vi "数据包生成.vi"(0 "状态：":string, 1 "旋转角度：":dbl, 2 "脉冲频率：":dbl, 3 "旋转方向：":bool, 4 "帧头：":string) -> (5 "数据包":string)   [LabVIEW 2018]
panel:
  out "旋转频率字符串":string
  out "旋转频率长度字符串":string
  out "旋转角度":string
  out "旋转角度字长字符串":string
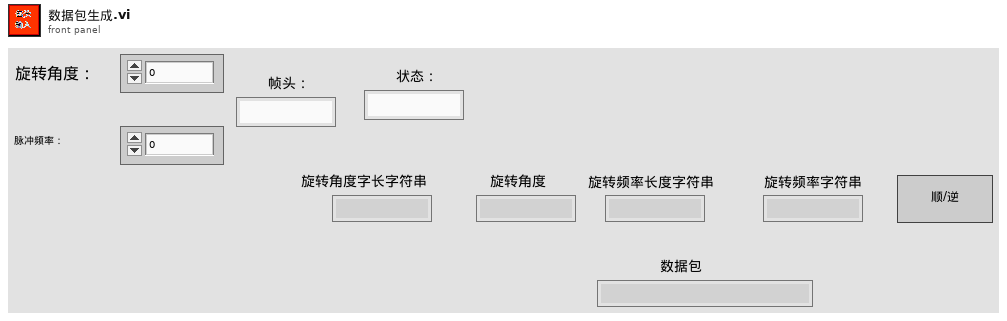
[diagram p1: front panel]
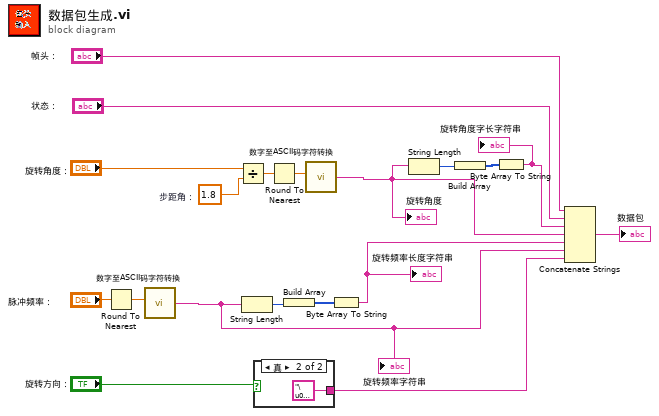
[diagram p0: block diagram]
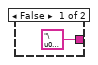
[diagram p2: hidden frame]
diagram:
  w19 = 1.8  # 步距角：
  n1 = Round To Nearest(number="脉冲频率：") -> (nearest integer value=w7:dbl)
  n2 = call "数字至ASCII码字符转换.vi"("数字"=w7) -> ("ASCII码字符串"=w1:string)  [unwired: 3 in]
  "旋转频率字符串" <- w1
  n3 = Divide(x="旋转角度：", y=w19) -> (x/y=w17:dbl)
  n4 = String Length(string=w1) -> (length=w9:i32)
  n5 = case shown="真" "旋转方向：" {
    tunnel: ["\u0000" "\u0001"] -> w6
    frame False {
    }
    frame True {
    }
  }
  n6 = Round To Nearest(number=w17) -> (nearest integer value=w8:dbl)
  n7 = Build Array(w9) -> (w10:i32[])
  n8 = call "数字至ASCII码字符转换.vi"("数字"=w8) -> ("ASCII码字符串"=w2:string)  [unwired: 3 in]
  "旋转角度" <- w2
  n9 = Byte Array To String(unsigned byte array=w10) -> (string=w5:string)
  "旋转频率长度字符串" <- w5
  n10 = String Length(string=w2) -> (length=w12:i32)
  n11 = Build Array(w12) -> (w11:i32[])
  n12 = Byte Array To String(unsigned byte array=w11) -> (string=w4:string)
  "旋转角度字长字符串" <- w4
  n13 = Concatenate Strings("帧头：", "状态：", w4, w2, w5, w1, w6) -> (→"数据包":string)
